vi "create.vi"(8 "error in (no error)":errorcluster, 9 "name":string, 10 "Image Type":T1 items=["Grayscale (U8)", "Grayscale (I16)", "Grayscale (SGL)", "Complex (CSG)", "RGB (U32)", "HSL (U32)", "RGB (U64)", "Grayscale (U16)"], 11 "Image in":refnum<class "Image.lvclass">) -> (0 "error out":errorcluster, 3 "Image out":refnum<class "Image.lvclass">)   [LabVIEW 2010, in "Image.lvclass"]
uses:
  Image.lvclass
  ErrorController/ErrorController/class_data.vi
  ErrorController/ErrorController/ErrorController.lvclass
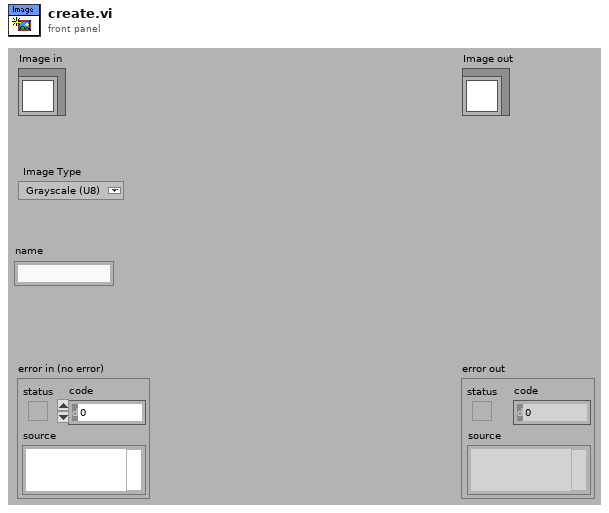
[diagram p1: front panel]
types:
  T1 = typedef "Image Type" = u32
  T2 = typedef "Image.lvclass/storage_mode.ctl" = enum16{"RAM", "disk"}
  T3 = typedef "IMAQ Image.ctl" = refnum<image>
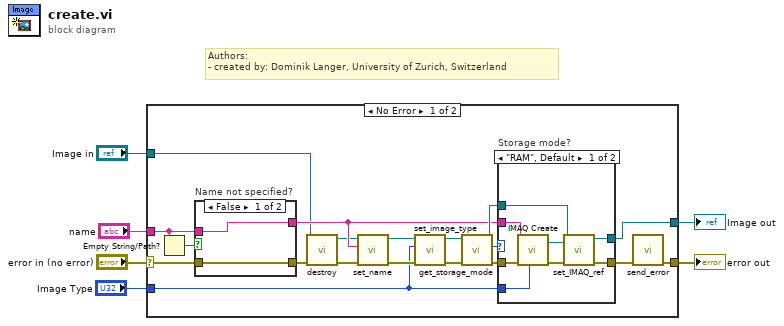
[diagram p0: block diagram]
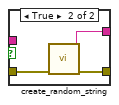
[diagram p3: hidden frame]
diagram:
  # "Authors: \n- created by: Dominik Langer, University of Zurich, Switzerland"
  n1 = case shown="No Error" "error in (no error)" {
    selector: "error in (no error)" -> [w24 w42]
    tunnel: [w8 w42] -> w5
    tunnel: [w25 w41] -> w3
    tunnel: "Image in" -> [w10 w41]
    tunnel: "Image Type" -> [w13 _]
    tunnel: "name" -> [w22 _]
    frame No Error {
      n2 = Empty String/Path?(string/path=w22) -> (empty?=w23:bool)
      n3 = case "Name not specified?" shown="False" w23 {
        tunnel: [w37 w40] -> w14
        tunnel: [w36 w39] -> w11
        tunnel: w24 -> [w36 w38]
        tunnel: w22 -> [w37 _]
        frame False {
        }
        frame True {
          n4 = call "create_random_string.vi"("error in (no error)"=w38) -> ("error out"=w39:errorcluster, "random string"=w40:string)  [unwired: 1 in, 8 out]
        }
      }
      n5 = call-dynamic "destroy.vi"("error in (no error)"=w11, "Image in"=w10) -> ("error out"=w12:errorcluster, "Image out"=w9:refnum<class "Image.lvclass">)  [unwired: 8 in]
      n6 = call-dynamic "set_name.vi"("error in (no error)"=w12, "name"=w14, "Image.lvclass in"=w9) -> ("error out"=w16:errorcluster, "Image.lvclass out"=w15:refnum<class "Image.lvclass">)  [unwired: 7 out]
      n7 = call-dynamic "set_image_type.vi"("error in (no error)"=w16, "Image Type"=w13, "Image.lvclass in"=w15) -> ("error out"=w18:errorcluster, "Image.lvclass out"=w17:refnum<class "Image.lvclass">)  [unwired: 7 out]
      n8 = call-dynamic "get_storage_mode.vi"("error in (no error)"=w18, "Image.lvclass in"=w17) -> ("error out"=w20:errorcluster, "storage mode"=w19:T2, "Image.lvclass out"=w21:refnum<class "Image.lvclass">)  [unwired: 7 out]
      n9 = case "Storage mode?" shown="\"RAM\", Default" w19 {
        tunnel: [w33 w35] -> w7
        tunnel: [w32 w34] -> w25
        tunnel: w14 -> [w29 _]
        tunnel: w21 -> [w28 w34]
        tunnel: w20 -> [w27 w35]
        tunnel: w13 -> [w26 _]
        frame "RAM", Default {
          n10 = call "IMAQ Create"("Image Name"=w29, "Image Type"=w26, "error in (no error)"=w27) -> ("New Image"=w31:T3, "error out"=w30:errorcluster)  [unwired: 1 in, 1 out]
          n11 = call-dynamic "set_IMAQ_ref.vi"("error in (no error)"=w30, "Image"=w31, "Image.lvclass in"=w28) -> ("error out"=w33:errorcluster, "Image.lvclass out"=w32:refnum<class "Image.lvclass">)  [unwired: 7 out]
        }
        frame "disk" {
        }
      }
      n12 = call "send_error.vi"("error in (no error)"=w7) -> ("error out"=w8:errorcluster)  [unwired: 10 in]
    }
    frame Error {
    }
  }
  "error out" <- w5
  "Image out" <- w3
